vi "ESP301 GetPos.vi"(5 "Axe Inv":bool, 6 "Input Units":i8(ring) items=["mm", "ps"], 7 "ESP301Ref":T1, 8 "error in":errorcluster, 9 "Axis":i8(ring)=1 items=["Axis 1"=1, "Axis 2"=2, "Axis 3"=3], 11 "VISA Rsrc":refnum<visa-resource-name>="GPIB0::7::INSTR") -> (0 "error out":errorcluster, 2 "Pos Out":dbl=0.5)   [LabVIEW 2019]
uses:
  <userlib>/ESP300/ESP300 GotoState.ctl
  <userlib>/GenProg/WritebyRefNum.vi
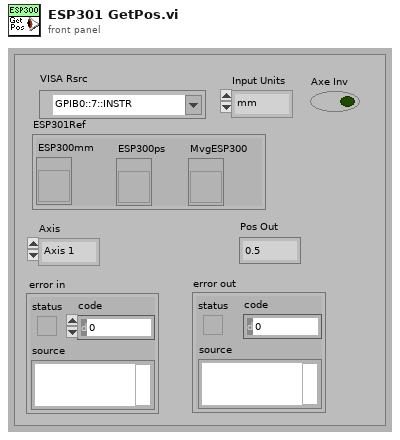
[diagram p1: front panel]
types:
  T1 = cluster{"ESP300mm":refnum<vi>, "ESP300ps":refnum<vi>, "MvgESP300":refnum<vi>}
  T2 = typedef "ESP300 GotoState.ctl" = enum16{"send command", "read position", "check status", "end"}
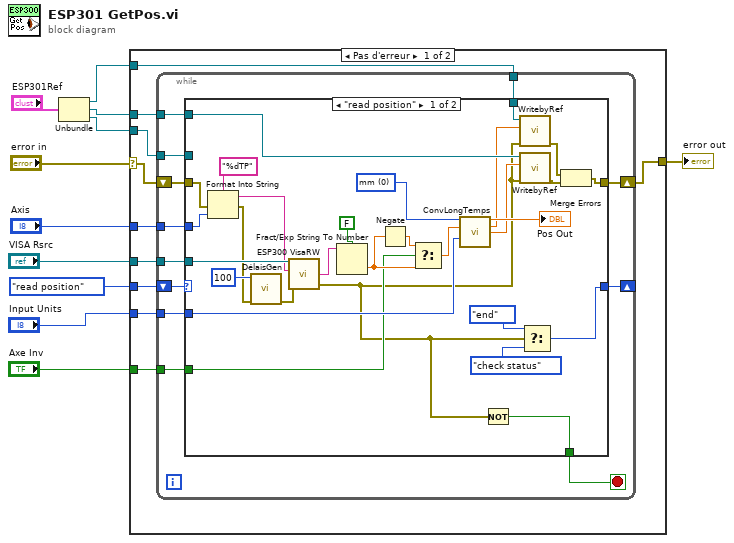
[diagram p0: block diagram]
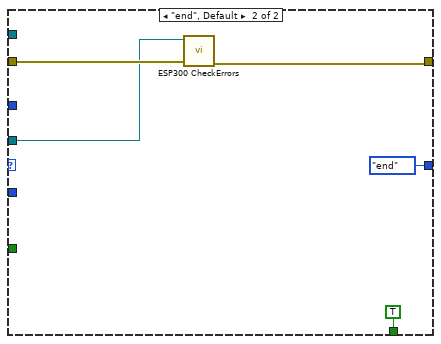
[diagram p2: hidden frame]
diagram:
  n1 = Unbundle("ESP301Ref") -> ("ESP300mm"=w2:refnum<vi>, "ESP300ps"=w4:refnum<vi>, "MvgESP300"=w3:refnum<vi>)
  n2 = case shown="Pas d'erreur" "error in" {
    selector: "error in" -> [w19 w68]
    tunnel: "Axis" -> [w21 _]
    tunnel: [w18 w68] -> w9
    tunnel: ESP300_GotoState."read position" ("Énum") -> [w20 _]
    tunnel: "VISA Rsrc" -> [w17 _]
    tunnel: w3 -> [w16 _]
    tunnel: "Input Units" -> [w15 _]
    tunnel: w2 -> [w14 _]
    tunnel: w4 -> [w13 _]
    tunnel: "Axe Inv" -> [w12 _]
    frame No Error {
      n3 = while {
        tunnel: w21 -> [w33]
        shift-right: [w29] -> w18
        shift-left: w19 -> [w31]
        tunnel: w17 -> [w30]
        shift-right: [w27] -> _
        shift-left: w20 -> [w32]
        tunnel: w16 -> [w26]
        tunnel: w15 -> [w25]
        tunnel: w14 -> [w24]
        tunnel: w13 -> [w23]
        tunnel: w12 -> [w22]
        stop <- w28 stop-if-true
        n4 = case shown="\"read position\"" w32 {
          tunnel: w33 -> [w60 _]
          tunnel: w31 -> [w59 w65]
          tunnel: w30 -> [w62 w63]
          tunnel: [w48 w64] -> w29
          tunnel: [w34 TRUE] -> w28
          tunnel: [w53 ESP300_GotoState."end" ("Énum")] -> w27
          tunnel: w26 -> [_ _]
          tunnel: w25 -> [w40 _]
          tunnel: w24 -> [w46 _]
          tunnel: w23 -> [w45 _]
          tunnel: w22 -> [w36 _]
          frame "read position" {
            w44 = i8 0 items=["mm", "ps"] ("Input Units")
            n5 = Format Into String(format string="%dTP", error in=w59, w60) -> (resulting string=w58:string, error out=w50:errorcluster)  [unwired: 1 in]
            n6 = call "DélaisGen.vi"("error in (no error)"=w50, "ms To Wait"=u32 100 ("milliseconds to wait")) -> ("error out"=w51:errorcluster)  [unwired: 9 in]
            n7 = call <userlib>:"ESP300 VisaRW.vi"("error in (no error)"=w51, "ChaineCom"=w58, "VISA Rsrc"=w62) -> ("error out"=w35:errorcluster, "ChaineRep"=w57:string)  [unwired: 4 in, 2 out]
            n8 = Fract/Exp String To Number(use system decimal point (T)=FALSE ("utiliser le séparateur décimal du système (V)"), string=w57) -> (number=w38:dbl)  [unwired: 2 in, 1 out]
            n9 = Negate(x=w38) -> (-x=w39:dbl)
            n10 = Select(t=w39, s=w36, f=w38) -> (s? t:f=w37:dbl)
            n11 = call <userlib>:"ConvLongTemps.vi"("Input Units"=w44, "Units Input"=w37, "Output Units"=w40) -> ("Units Output"=→"Pos Out":dbl, "Units mm"=w42:dbl, "Units ps"=w41:dbl)  [unwired: 9 in, 1 out]
            n12 = Not(x=w35) -> (.not. x?=w34:bool)
            n13 = call-poly <userlib>:"WritebyRef.vi"("error in"=w35, "Valeur"=w42, "Control Ref"=w46) -> ("error out"=w47:errorcluster)  [unwired: 8 in]
            n14 = call-poly <userlib>:"WritebyRef.vi"("error in"=w35, "Valeur"=w41, "Control Ref"=w45) -> ("error out"=w49:errorcluster)  [unwired: 8 in]
            n15 = Select(t=ESP300_GotoState."end" ("Énum"), s=w35, f=ESP300_GotoState."check status" ("Énum")) -> (s? t:f=w53:T2)
            n16 = Merge Errors(w47, w49) -> (w48:errorcluster)
          }
          frame "end", Default {
            n17 = call <userlib>:"ESP300 CheckErrors.vi"("error in (no error)"=w65, "Ressource VISA In"=w63) -> ("error out"=w64:errorcluster)  [unwired: 4 in, 3 out]
          }
        }
      }
    }
    frame Error {
    }
  }
  "error out" <- w9
